vi "Create.vi"(8 "error in (no error)":errorcluster, 10 "Shot":i32, 11 "Name":string) -> (0 "error out":errorcluster, 3 "Tree out":refnum<class "Tree.lvclass">)   [LabVIEW 2012, in "MDSplus.lvlib" / "Tree.lvclass"]
uses:
  <vilib>/MDSplus/Classes/Tree_Class/Tree.lvclass
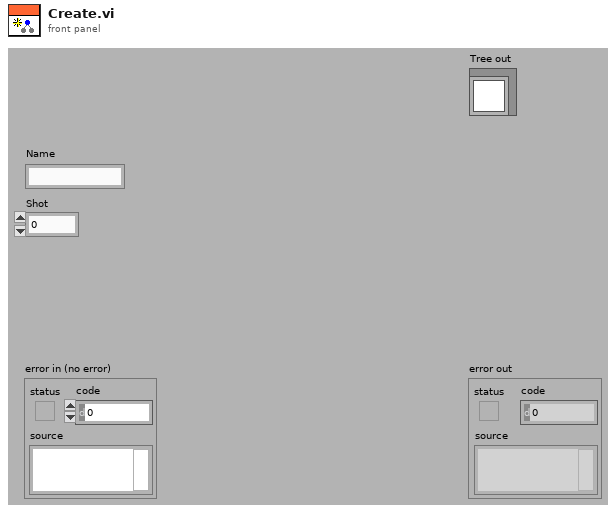
[diagram p1: front panel]
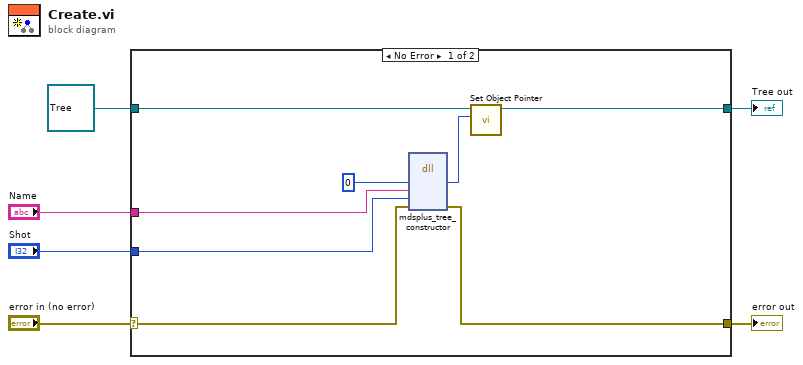
[diagram p0: block diagram]
diagram:
  n1 = case shown="No Error" "error in (no error)" {
    selector: "error in (no error)" -> [w8 w16]
    tunnel: [w7 w16] -> w5
    tunnel: [w10 w15] -> w3
    tunnel: refnum<class "Tree.lvclass"> refnum ("Tree in") -> [w11 w15]
    tunnel: "Name" -> [w13 _]
    tunnel: "Shot" -> [w12 _]
    frame No Error {
      n2 = dll-call lib="MDSobjectsLVShr" fn="mdsplus_tree_constructor"("lvTreePtr"=i64 0, "nameIn"=w13, "shotIn"=w12, "error"=w8) -> ("lvTreePtr"=w9:i64, "error"=w7:errorcluster)  [unwired: 6 in, 2 out]
      n3 = call-dynamic "Set Object Pointer.vi"("Object Pointer"=w9, "Tree in"=w11) -> ("Tree out"=w10:refnum<class "Tree.lvclass">)  [unwired: 9 in]
    }
    frame Error {
    }
  }
  "error out" <- w5
  "Tree out" <- w3
